vi "start.vi"(8 "error in":errorcluster, 10 "queue to parent":refnum<queue>, 11 "communicator in":refnum<class "communicator.lvclass">) -> (0 "error out":errorcluster, 3 "communicator out":refnum<class "communicator.lvclass">)   [LabVIEW 2015, in "communicator.lvclass"]
uses:
  communicator.lvclass
  message/communicator message.lvclass
  communicator.lvclass/communicator.ctl
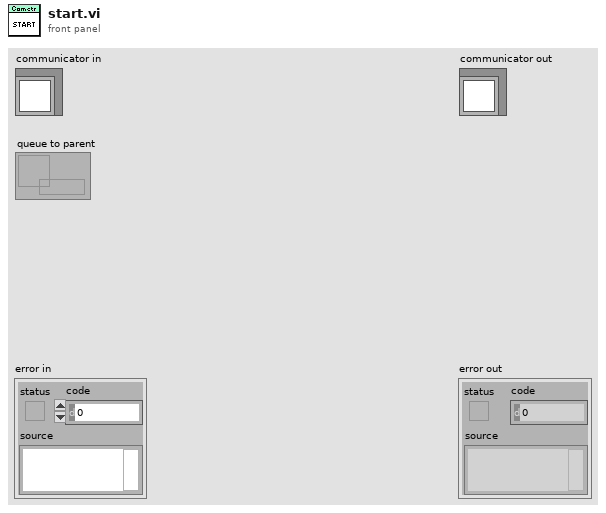
[diagram p1: front panel]
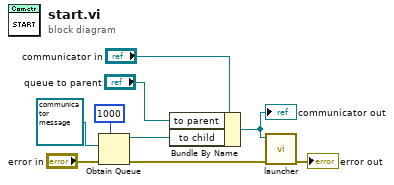
[diagram p0: block diagram]
diagram:
  n1 = Obtain Queue(max queue size (-1, unlimited)=1000, element data type=refnum<class "communicator message.lvclass"> refnum ("communicator message.lvclass"), error in (no error)="error in") -> (queue out=w6:refnum<queue>, error out=w5:errorcluster)  [unwired: 2 in, 1 out]
  n2 = Bundle By Name(cluster="communicator in", "to parent"="queue to parent", "to child"=w6) -> (w3:refnum<class "communicator.lvclass">)
  "communicator out" <- w3
  n3 = call "launcher.vi"("error in"=w5, "communicator in"=w3) -> ("error out"=→"error out":errorcluster)  [unwired: 9 in]
